vi "file name prefix.vi"(8 "Fast sweep settings":T2={"Update rate (Hz)"=200.0, "Start F, Hz"=50000.0, "Stop F"=1000000.0, "Number of points"=100000, "Amplitude"=2.1, "Init&amplitude"=TRUE, "IF"=1000.0, "Time constant"=0.003} {"IF" format="%#_6p"; "Amplitude" min=0.0 max=2.5; "Number of points" format="%.0p"; "Stop F" format="%#_6p"; "Start F, Hz" format="%#_6p"; "Update rate (Hz)" format="%0.2f"}, 10 "Magn Field (T)":dbl, 11 "temperature":dbl=1.9) -> (0 "minutes/sweep":dbl=8.333333333333334, 1 "kHz/second":dbl=1.9, 2 "file name prefix":string, 3 "filename cluster OUT":T1={"mmddyy (str)"="", "counter (str)"="", "to F (kHz)"=0.0, "from F (kHz)"=0.0, "temperature (K)"=0.0, "date/time string"="", "time stamp"=timestamp(19856294.882018566 s since 1904-01-01), "base name"="", "temperature (str)"="", "from F (str)"="", "to F (str)"="", "format"=enum."no date string", "power (V)"=0.0, "power (str) "="", "Magn Field (T)"=0.0, "Magn Field (str)"=""})   [LabVIEW 2016]
uses:
  resonant_ultrasound/Libraries/RUS/Controls/Sweep settings.ctl
  file -- scan filename.ctl
  file -- scan filename action.ctl
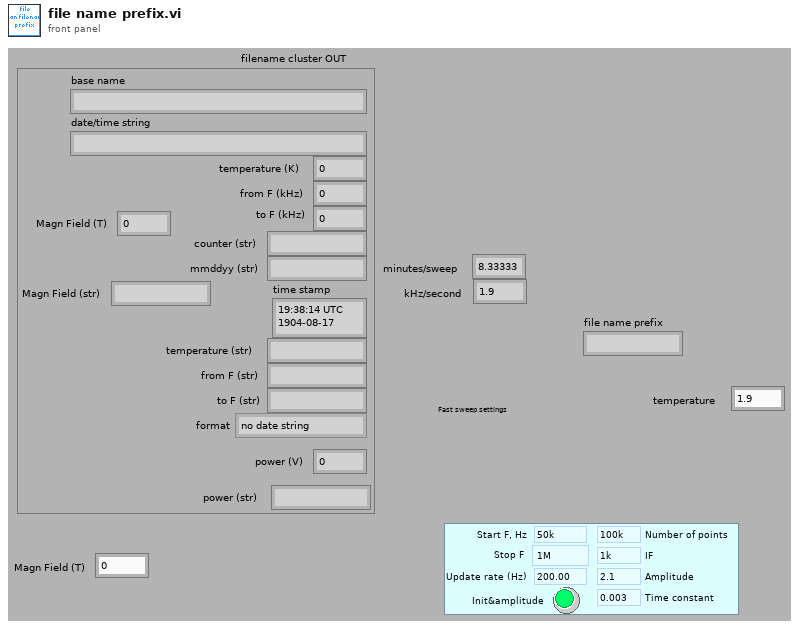
[diagram p1: front panel]
types:
  T1 = typedef "file -- scan filename.ctl" = cluster{"mmddyy (str)":string, "counter (str)":string, "to F (kHz)":dbl, "from F (kHz)":dbl, "temperature (K)":dbl, "date/time string":string, "time stamp":timestamp, "base name":string, "temperature (str)":string, "from F (str)":string, "to F (str)":string, "format":enum16{"no date string", "with date string"}, "power (V)":dbl, "power (str) ":string, "Magn Field (T)":dbl, "Magn Field (str)":string}
  T2 = typedef "Sweep settings.ctl" = cluster{"Update rate (Hz)":dbl, "Start F, Hz":dbl, "Stop F":dbl, "Number of points":i32, "Amplitude":dbl, "Init&amplitude":bool, "IF":dbl, "Time constant":dbl}
  T3 = typedef "file -- scan filename action.ctl" = enum16{"prefix base name", "datestring regexp", "parse datestring", "datestring", "filename regexp", "parse filename", "datestring regexp (no brackets)", "suffix base name"}
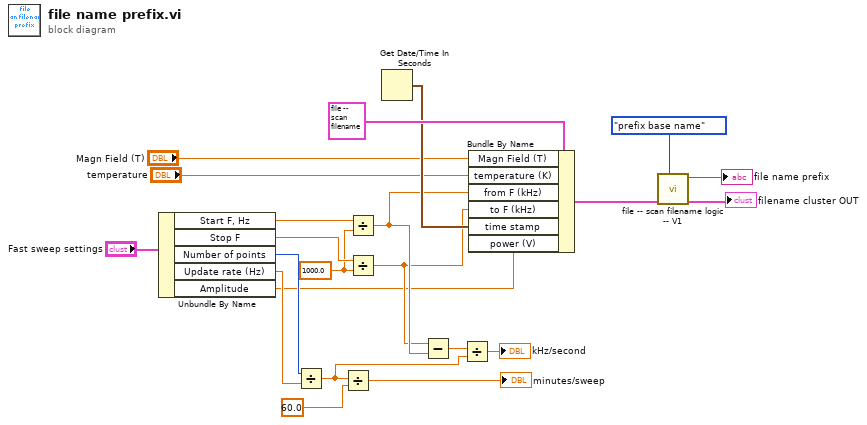
[diagram p0: block diagram]
diagram:
  w20 = 1000.0 ("y")
  n1 = Unbundle By Name("Fast sweep settings") -> ("Start F, Hz"=w22:dbl, "Stop F"=w21:dbl, "Number of points"=w19:i32, "Update rate (Hz)"=w18:dbl, "Amplitude"=w2:dbl)
  n2 = Divide(x=w19, y=w18) -> (x/y=w15:dbl)
  n3 = Divide(x=w15, y=60.0) -> (x/y=→"minutes/sweep":dbl)
  n4 = Divide(x=w22, y=w20) -> (x/y=w7:dbl)
  n5 = Divide(x=w21, y=w20) -> (x/y=w6:dbl)
  n6 = Get Date/Time In Seconds() -> (seconds since 1Jan1904=w9:timestamp)
  n7 = Subtract(x=w6, y=w7) -> (x-y=w16:dbl)
  n8 = Divide(x=w16, y=w15) -> (x/y=→"kHz/second":dbl)
  n9 = Bundle By Name(cluster=T1 {"mmddyy (str)"="", "counter (str)"="", "to F (kHz)"=0.0, "from F (kHz)"=0.0, "temperature (K)"=0.0, "date/time string"="", "time stamp"=timestamp(19856294.882018566 s since 1904-01-01), "base name"="", "temperature (str)"="", "from F (str)"="", "to F (str)"="", "format"=enum."no date string", "power (V)"=0.0, "power (str) "="", "Magn Field (T)"=0.0, "Magn Field (str)"=""} ("scan filename IN"), "Magn Field (T)"="Magn Field (T)", "temperature (K)"="temperature", "from F (kHz)"=w7, "to F (kHz)"=w6, "time stamp"=w9, "power (V)"=w2) -> (w5:T1)
  n10 = call "file -- scan filename logic -- V1.vi"("scan fileneme action"=file_--_scan_filename_action."prefix base name" ("scan filename action"), "scan filename IN"=w5) -> ("scan filename OUT"=→"filename cluster OUT":T1, "string OUT"=→"file name prefix":string)  [unwired: 7 in, 1 out]
